vi "Decode_RAW_to_DEC.vi"(1 "Read TTL status":bool, 2 "read buffer":string) -> (0 "DEC SGL output":sgl[][](array[numeric]))   [LabVIEW 2016]
panel:
  out "transposed array":sgl[][](array[numeric])
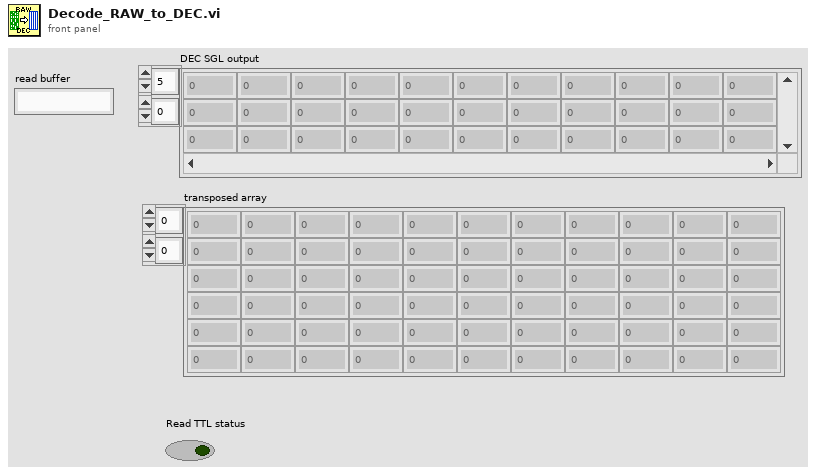
[diagram p1: front panel]
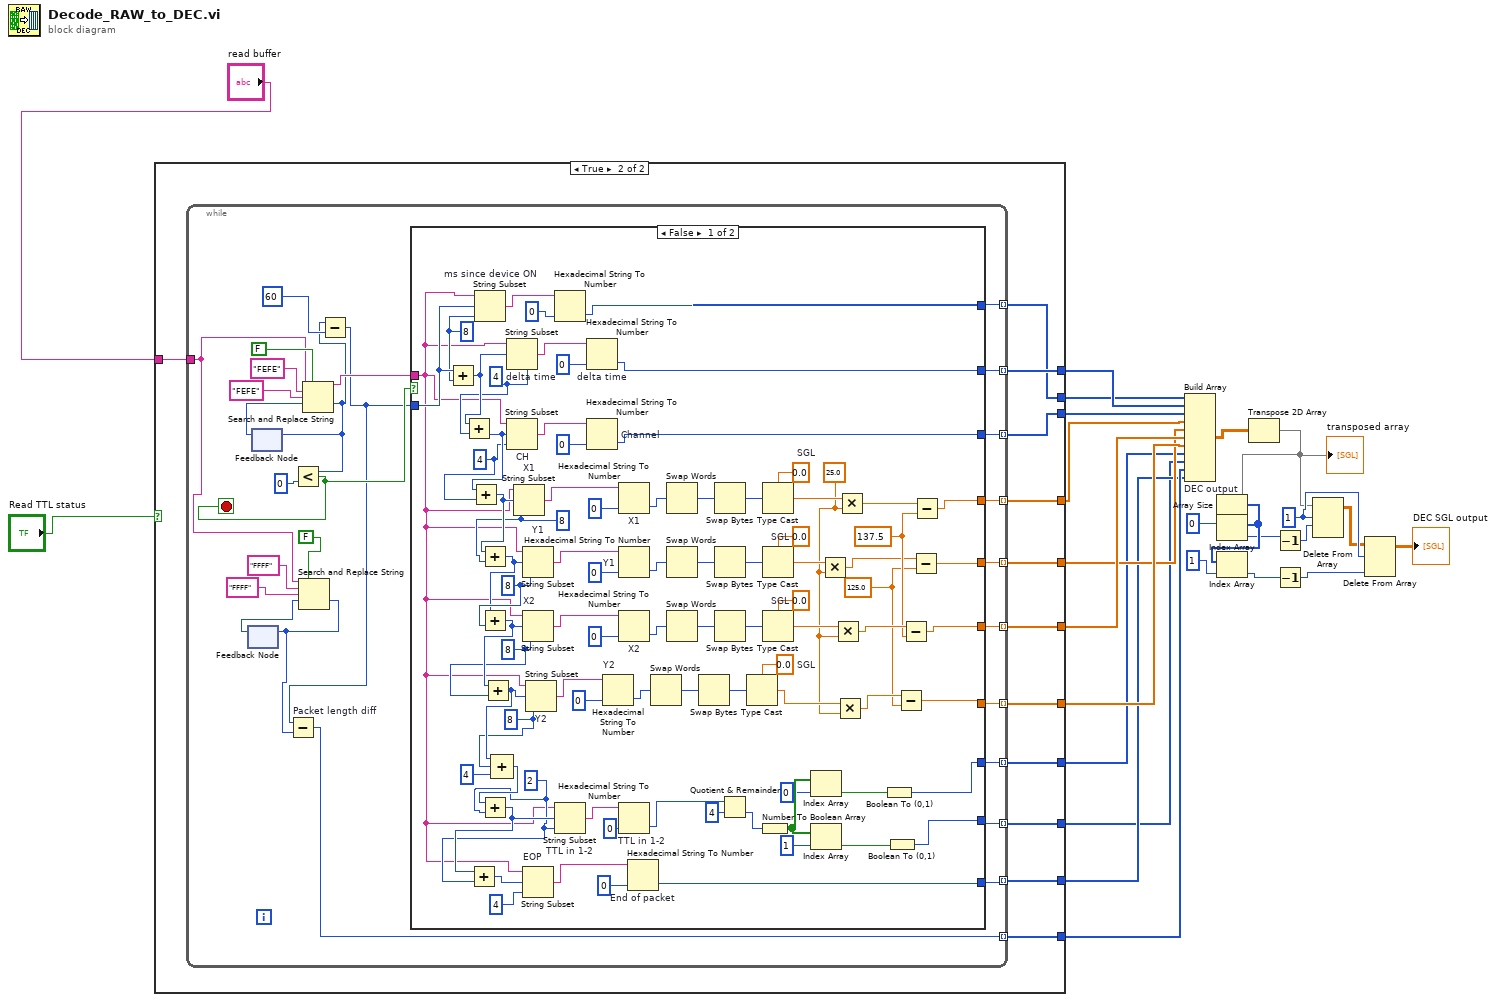
[diagram p0: block diagram]
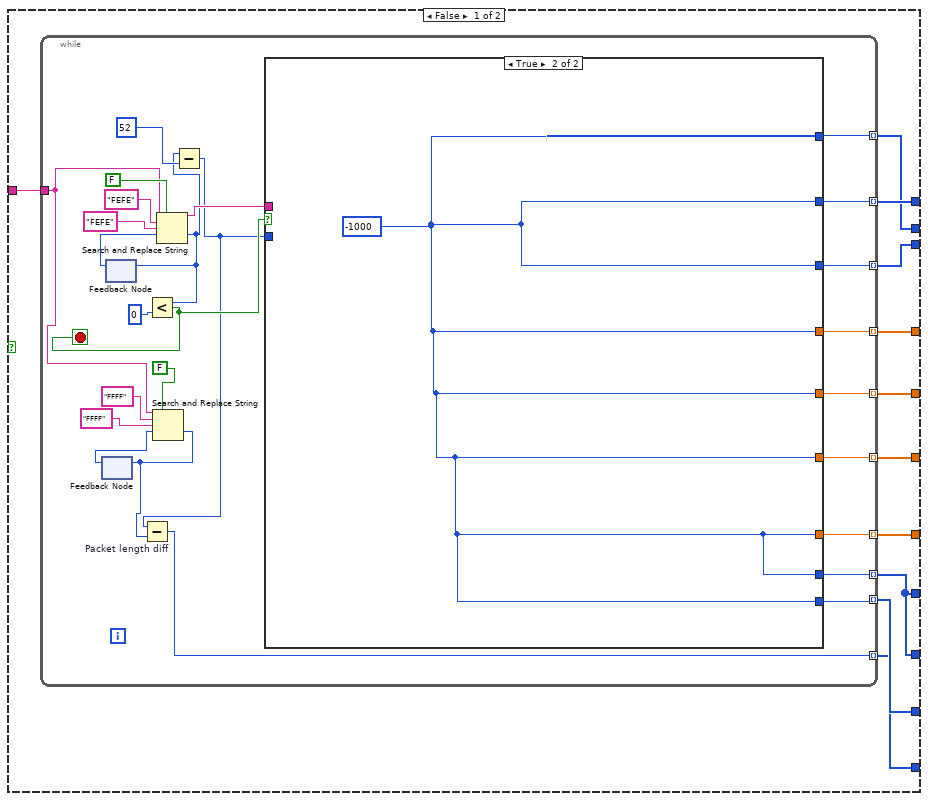
[diagram p2: hidden frame]
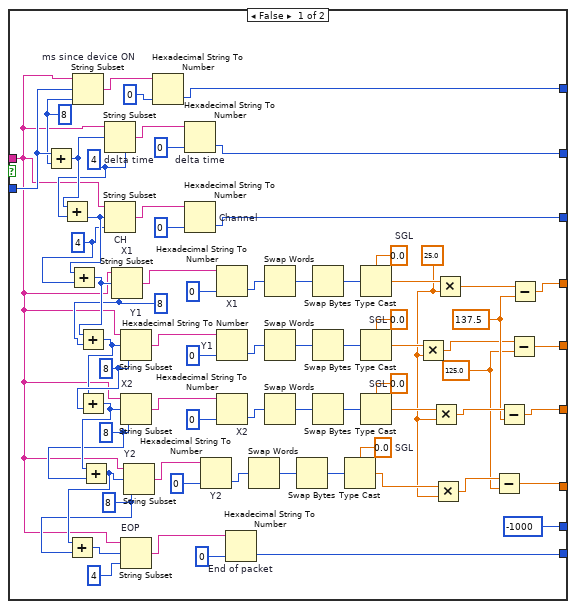
[diagram p3: hidden frame]
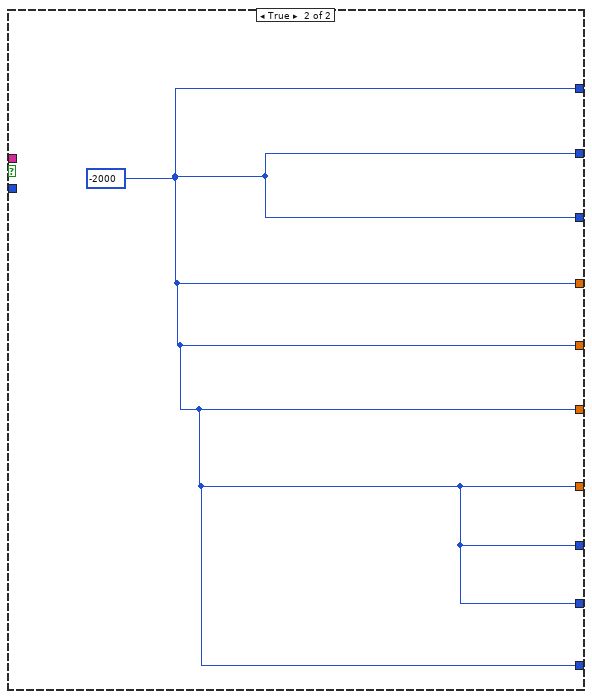
[diagram p4: hidden frame]
diagram:
  w21 = 1 ("length")
  n1 = case shown="True" "Read TTL status" {
    tunnel: [w36 w144] -> w14
    tunnel: [w35 w143] -> w13
    tunnel: [w34 w142] -> w12
    tunnel: [w33 w141] -> w11
    tunnel: [w32 w140] -> w10
    tunnel: [w31 w139] -> w9
    tunnel: [w30 w138] -> w8
    tunnel: "read buffer" -> [w29 w137]
    tunnel: [w28 w136] -> w3
    tunnel: [w27 w135] -> w4
    tunnel: [w26 w134] -> w2
    tunnel: [w26 w133] -> w1
    frame False {
      n2 = while {
        tunnel: w29 -> [w44]
        tunnel: [w56] -> w30 mode=indexing
        tunnel: [w54] -> w31 mode=indexing
        tunnel: [w53] -> w32 mode=indexing
        tunnel: [w52] -> w33 mode=indexing
        tunnel: [w51] -> w34 mode=indexing
        tunnel: [w50] -> w35 mode=indexing
        tunnel: [w49] -> w36 mode=indexing
        tunnel: [w48] -> w28 mode=indexing
        tunnel: [w41] -> w27 mode=indexing
        tunnel: [w37] -> w26 mode=indexing
        stop <- w55 stop-if-true
        n3 = feedback #1() -> (w43:i32)  [unwired: 1 in]
        n4 = feedback #2() -> (w59:i32)  [unwired: 1 in]
        n5 = Search and Replace String(replace all?=FALSE ("replace all? (F)"), input string=w44, search string="FFFF", replace string="FFFF" ("replace string (\"\")"), offset=w43) -> (offset past replacement=w40:i32)  [unwired: 3 in, 3 out]
        n6 = feedback-in #1(w40) -> ()
        n7 = Search and Replace String(replace all?=FALSE ("replace all? (F)"), input string=w44, search string="FEFE", replace string="FEFE" ("replace string (\"\")"), offset=w59) -> (result string=w57:string, offset past replacement=w39:i32)  [unwired: 3 in, 2 out]
        n8 = feedback-in #2(w39) -> ()
        n9 = Less?(x=w39, y=0) -> (x < y?=w55:bool)
        n10 = Subtract(x=w39, y=52) -> (x-y=w38:i32)
        n11 = Subtract "Packet length diff"(x=w38, y=w40) -> (x-y=w41:i32)
        n12 = case shown="True" w55 {
          tunnel: w57 -> [w115 _]
          tunnel: [w112 w132] -> w56
          tunnel: w38 -> [w131 _]
          tunnel: [w109 w132] -> w54
          tunnel: [w106 w132] -> w53
          tunnel: [w73 w132] -> w52
          tunnel: [w68 w132] -> w51
          tunnel: [w71 w132] -> w50
          tunnel: [w66 w132] -> w49
          tunnel: [w75 w132] -> w48
          tunnel: [-1000 w132] -> w37
          frame False {
            w64 = sgl 125.0 ("Half-height of the sensor board")
            w69 = sgl 137.5 ("Half-width of the sensor board")
            w74 = sgl 25.0 ("y")
            w81 = sgl 0.0  # SGL
            w88 = sgl 0.0  # SGL
            w95 = sgl 0.0  # SGL
            w101 = sgl 0.0  # SGL
            w117 = 8 ("length (rest)")
            w120 = 8 ("length (rest)")
            w123 = 8 ("length (rest)")
            w124 = 8 ("length (rest)")
            w126 = 4 ("length (rest)")
            w128 = 4 ("length (rest)")
            w130 = 8 ("length (rest)")
            n13 = Add(x=w131, y=w130) -> (x+y=w129:i32)
            n14 = Add(x=w129, y=w128) -> (x+y=w127:i32)
            n15 = Add(x=w127, y=w126) -> (x+y=w125:i32)
            n16 = String Subset "ms since device ON"(string=w115, offset (0)=w131, length (rest)=w130) -> (substring=w114:string)
            n17 = Add(x=w125, y=w124) -> (x+y=w122:i32)
            n18 = Add(x=w122, y=w123) -> (x+y=w121:i32)
            n19 = Add(x=w121, y=w120) -> (x+y=w118:i32)
            n20 = Add(x=w118, y=w117) -> (x+y=w119:i32)
            n21 = String Subset "delta time"(string=w115, offset (0)=w129, length (rest)=w128) -> (substring=w110:string)
            n22 = String Subset "CH"(string=w115, offset (0)=w127, length (rest)=w126) -> (substring=w107:string)
            n23 = String Subset "X1"(string=w115, offset (0)=w125, length (rest)=w124) -> (substring=w105:string)
            n24 = String Subset "Y1"(string=w115, offset (0)=w122, length (rest)=w123) -> (substring=w93:string)
            n25 = String Subset "X2"(string=w115, offset (0)=w121, length (rest)=w120) -> (substring=w86:string)
            n26 = String Subset "EOP"(string=w115, offset (0)=w119, length (rest)=4 ("length (rest)")) -> (substring=w76:string)
            n27 = String Subset "Y2"(string=w115, offset (0)=w118, length (rest)=w117) -> (substring=w79:string)
            n28 = Hexadecimal String To Number ("ms since ON")(string=w114, default (0uL)=u32 0 ("default (0 U32)")) -> (number=w112:u32)  [unwired: 1 in, 1 out]
            n29 = Hexadecimal String To Number "delta time"(string=w110, default (0uL)=u32 0 ("default (0 U32)")) -> (number=w109:u32)  [unwired: 1 in, 1 out]
            n30 = Hexadecimal String To Number "Channel"(string=w107, default (0uL)=u32 0 ("default (0 U32)")) -> (number=w106:u32)  [unwired: 1 in, 1 out]
            n31 = Hexadecimal String To Number "Y2"(string=w79, default (0uL)=u32 0 ("default (0 U32)")) -> (number=w83:u32)  [unwired: 1 in, 1 out]
            n32 = Hexadecimal String To Number "X1"(string=w105, default (0uL)=u32 0 ("default (0 U32)")) -> (number=w103:u32)  [unwired: 1 in, 1 out]
            n33 = Hexadecimal String To Number "Y1"(string=w93, default (0uL)=u32 0 ("default (0 U32)")) -> (number=w97:u32)  [unwired: 1 in, 1 out]
            n34 = Hexadecimal String To Number "X2"(string=w86, default (0uL)=u32 0 ("default (0 U32)")) -> (number=w90:u32)  [unwired: 1 in, 1 out]
            n35 = Hexadecimal String To Number "End of packet"(string=w76, default (0uL)=u32 0 ("default (0 U32)")) -> (number=w75:u32)  [unwired: 1 in, 1 out]
            n36 = Swap Words(1:w83) -> (0:w82:u32)
            n37 = Swap Words(1:w103) -> (0:w102:u32)
            n38 = Swap Words(1:w97) -> (0:w96:u32)
            n39 = Swap Words(1:w90) -> (0:w89:u32)
            n40 = Swap Bytes(anything=w82) -> (byte swapped=w80:u32)
            n41 = Swap Bytes(anything=w102) -> (byte swapped=w100:u32)
            n42 = Swap Bytes(anything=w96) -> (byte swapped=w94:u32)
            n43 = Swap Bytes(anything=w89) -> (byte swapped=w87:u32)
            n44 = Type Cast(type=w81, x=w80) -> (*(type *) &x=w78:sgl)
            n45 = Type Cast(type=w101, x=w100) -> (*(type *) &x=w99:sgl)
            n46 = Type Cast(type=w95, x=w94) -> (*(type *) &x=w92:sgl)
            n47 = Type Cast(type=w88, x=w87) -> (*(type *) &x=w85:sgl)
            n48 = Multiply(x=w92, y=w74) -> (x*y=w67:sgl)
            n49 = Multiply(x=w85, y=w74) -> (x*y=w70:sgl)
            n50 = Multiply(x=w78, y=w74) -> (x*y=w65:sgl)
            n51 = Multiply(x=w99, y=w74) -> (x*y=w72:sgl)
            n52 = Subtract(x=w65, y=w64) -> (x-y=w66:sgl)
            n53 = Subtract(x=w70, y=w69) -> (x-y=w71:sgl)
            n54 = Subtract(x=w67, y=w64) -> (x-y=w68:sgl)
            n55 = Subtract(x=w72, y=w69) -> (x-y=w73:sgl)
          }
          frame True {
            w132 = -1000
          }
        }
      }
    }
    frame True {
      n56 = while {
        tunnel: w137 -> [w153]
        tunnel: [w165] -> w138 mode=indexing
        tunnel: [w163] -> w139 mode=indexing
        tunnel: [w162] -> w140 mode=indexing
        tunnel: [w161] -> w141 mode=indexing
        tunnel: [w160] -> w142 mode=indexing
        tunnel: [w159] -> w143 mode=indexing
        tunnel: [w158] -> w144 mode=indexing
        tunnel: [w157] -> w136 mode=indexing
        tunnel: [w150] -> w135 mode=indexing
        tunnel: [w145] -> w134 mode=indexing
        tunnel: [w146] -> w133 mode=indexing
        stop <- w164 stop-if-true
        n57 = feedback #3() -> (w152:i32)  [unwired: 1 in]
        n58 = feedback #4() -> (w168:i32)  [unwired: 1 in]
        n59 = Search and Replace String(replace all?=FALSE ("replace all? (F)"), input string=w153, search string="FFFF", replace string="FFFF" ("replace string (\"\")"), offset=w152) -> (offset past replacement=w149:i32)  [unwired: 3 in, 3 out]
        n60 = feedback-in #3(w149) -> ()
        n61 = Search and Replace String(replace all?=FALSE ("replace all? (F)"), input string=w153, search string="FEFE", replace string="FEFE" ("replace string (\"\")"), offset=w168) -> (result string=w166:string, offset past replacement=w148:i32)  [unwired: 3 in, 2 out]
        n62 = feedback-in #4(w148) -> ()
        n63 = Less?(x=w148, y=0) -> (x < y?=w164:bool)
        n64 = Subtract(x=w148, y=60) -> (x-y=w147:i32)
        n65 = Subtract "Packet length diff"(x=w147, y=w149) -> (x-y=w150:i32)
        n66 = case shown="False" w164 {
          tunnel: w166 -> [w182 _]
          tunnel: [w239 w256] -> w165
          tunnel: w147 -> [w255 _]
          tunnel: [w236 w256] -> w163
          tunnel: [w233 w256] -> w162
          tunnel: [w200 w256] -> w161
          tunnel: [w195 w256] -> w160
          tunnel: [w198 w256] -> w159
          tunnel: [w193 w256] -> w158
          tunnel: [w202 w256] -> w157
          tunnel: [w174 w256] -> w146
          tunnel: [w172 w256] -> w145
          frame False {
            w184 = 2 ("length (rest)")
            w191 = sgl 125.0 ("Half-height of the sensor board")
            w196 = sgl 137.5 ("Half-width of the sensor board")
            w201 = sgl 25.0 ("y")
            w208 = sgl 0.0  # SGL
            w215 = sgl 0.0  # SGL
            w222 = sgl 0.0  # SGL
            w228 = sgl 0.0  # SGL
            w189 = 8 ("length (rest)")
            w244 = 8 ("length (rest)")
            w247 = 8 ("length (rest)")
            w248 = 8 ("length (rest)")
            w250 = 4 ("length (rest)")
            w252 = 4 ("length (rest)")
            w254 = 8 ("length (rest)")
            n67 = Add(x=w255, y=w254) -> (x+y=w253:i32)
            n68 = Add(x=w253, y=w252) -> (x+y=w251:i32)
            n69 = Add(x=w251, y=w250) -> (x+y=w249:i32)
            n70 = String Subset "ms since device ON"(string=w182, offset (0)=w255, length (rest)=w254) -> (substring=w241:string)
            n71 = Add(x=w249, y=w248) -> (x+y=w246:i32)
            n72 = Add(x=w246, y=w247) -> (x+y=w245:i32)
            n73 = Add(x=w245, y=w244) -> (x+y=w190:i32)
            n74 = Compound Arithmetic op=ADD(w190, w189, 4 ("value")) -> (w186:i32)
            n75 = Add(x=w186, y=w184) -> (x+y=w185:i32)
            n76 = Add(x=w185, y=w184) -> (x+y=w243:i32)
            n77 = String Subset "delta time"(string=w182, offset (0)=w253, length (rest)=w252) -> (substring=w237:string)
            n78 = String Subset "CH"(string=w182, offset (0)=w251, length (rest)=w250) -> (substring=w234:string)
            n79 = String Subset "X1"(string=w182, offset (0)=w249, length (rest)=w248) -> (substring=w232:string)
            n80 = String Subset "Y1"(string=w182, offset (0)=w246, length (rest)=w247) -> (substring=w220:string)
            n81 = String Subset "X2"(string=w182, offset (0)=w245, length (rest)=w244) -> (substring=w213:string)
            n82 = String Subset "EOP"(string=w182, offset (0)=w243, length (rest)=4 ("length (rest)")) -> (substring=w203:string)
            n83 = String Subset "Y2"(string=w182, offset (0)=w190, length (rest)=w189) -> (substring=w206:string)
            n84 = Hexadecimal String To Number ("ms since ON")(string=w241, default (0uL)=u32 0 ("default (0 U32)")) -> (number=w239:u32)  [unwired: 1 in, 1 out]
            n85 = String Subset "TTL in 1-2"(string=w182, offset (0)=w185, length (rest)=w184) -> (substring=w188:string)
            n86 = Hexadecimal String To Number "delta time"(string=w237, default (0uL)=u32 0 ("default (0 U32)")) -> (number=w236:u32)  [unwired: 1 in, 1 out]
            n87 = Hexadecimal String To Number "Channel"(string=w234, default (0uL)=u32 0 ("default (0 U32)")) -> (number=w233:u32)  [unwired: 1 in, 1 out]
            n88 = Hexadecimal String To Number "Y2"(string=w206, default (0uL)=u32 0 ("default (0 U32)")) -> (number=w210:u32)  [unwired: 1 in, 1 out]
            n89 = Hexadecimal String To Number "X1"(string=w232, default (0uL)=u32 0 ("default (0 U32)")) -> (number=w230:u32)  [unwired: 1 in, 1 out]
            n90 = Hexadecimal String To Number "Y1"(string=w220, default (0uL)=u32 0 ("default (0 U32)")) -> (number=w224:u32)  [unwired: 1 in, 1 out]
            n91 = Hexadecimal String To Number "X2"(string=w213, default (0uL)=u32 0 ("default (0 U32)")) -> (number=w217:u32)  [unwired: 1 in, 1 out]
            n92 = Hexadecimal String To Number "TTL in 1-2"(string=w188, default (0uL)=u32 0 ("default (0 U32)")) -> (number=w180:u32)  [unwired: 1 in, 1 out]
            n93 = Hexadecimal String To Number "End of packet"(string=w203, default (0uL)=u32 0 ("default (0 U32)")) -> (number=w202:u32)  [unwired: 1 in, 1 out]
            n94 = Swap Words(1:w210) -> (0:w209:u32)
            n95 = Swap Words(1:w230) -> (0:w229:u32)
            n96 = Swap Words(1:w224) -> (0:w223:u32)
            n97 = Swap Words(1:w217) -> (0:w216:u32)
            n98 = Swap Bytes(anything=w209) -> (byte swapped=w207:u32)
            n99 = Swap Bytes(anything=w229) -> (byte swapped=w227:u32)
            n100 = Swap Bytes(anything=w223) -> (byte swapped=w221:u32)
            n101 = Swap Bytes(anything=w216) -> (byte swapped=w214:u32)
            n102 = Quotient & Remainder(x=w180, y=u32 4) -> (floor(x/y)=w179:u32)  [unwired: 1 out]
            n103 = Type Cast(type=w208, x=w207) -> (*(type *) &x=w205:sgl)
            n104 = Number To Boolean Array(number=w179) -> (Boolean array=w178:bool[])
            n105 = Type Cast(type=w228, x=w227) -> (*(type *) &x=w226:sgl)
            n106 = Type Cast(type=w222, x=w221) -> (*(type *) &x=w219:sgl)
            n107 = Type Cast(type=w215, x=w214) -> (*(type *) &x=w212:sgl)
            n108 = Index Array(array=w178, index=0) -> (element=w175:bool)
            n109 = Index Array(array=w178, index=1) -> (element=w173:bool)
            n110 = Multiply(x=w219, y=w201) -> (x*y=w194:sgl)
            n111 = Multiply(x=w212, y=w201) -> (x*y=w197:sgl)
            n112 = Multiply(x=w205, y=w201) -> (x*y=w192:sgl)
            n113 = Multiply(x=w226, y=w201) -> (x*y=w199:sgl)
            n114 = Boolean To (0,1)(Boolean=w175) -> (0, 1=w174:i16)
            n115 = Boolean To (0,1)(Boolean=w173) -> (0, 1=w172:i16)
            n116 = Subtract(x=w192, y=w191) -> (x-y=w193:sgl)
            n117 = Subtract(x=w197, y=w196) -> (x-y=w198:sgl)
            n118 = Subtract(x=w194, y=w191) -> (x-y=w195:sgl)
            n119 = Subtract(x=w199, y=w196) -> (x-y=w200:sgl)
          }
          frame True {
            w256 = -2000
          }
        }
      }
    }
  }
  n120 = Build Array "DEC output"(w8, w9, w10, w11, w12, w13, w14, w1, w2, w4, w3) -> (w15:sgl[][])
  n121 = Transpose 2D Array(2D array=w15) -> (transposed array=w16:sgl[][])
  "transposed array" <- w16
  n122 = Array Size(array=w16) -> (size(s)=w23:i32[])
  n123 = Index Array(array=w23, index=0) -> (element=w18:i32)
  n124 = Index Array(array=w23, index=1) -> (element=w24:i32)
  n125 = Decrement(x=w18) -> (x-1=w19:i32)
  n126 = Decrement(x=w24) -> (x-1=w25:i32)
  n127 = Delete From Array(array=w16, length=w21, index (row)=w19) -> (array with subset deleted=w20:sgl[][])  [unwired: 1 in, 1 out]
  n128 = Delete From Array(array=w20, length=w21, index (col)=w25) -> (array with subset deleted=→"DEC SGL output":sgl[][])  [unwired: 1 in, 1 out]
